vi "Update Online Status List.vi"(8 "error in (no error)":errorcluster, 10 "Online Status List":string[](array[string]), 11 "Chat Window Controller UI in":refnum<class "Chat Window Controller UI.lvclass">) -> (0 "error out":errorcluster, 3 "Chat Window Controller UI out":refnum<class "Chat Window Controller UI.lvclass">)   [LabVIEW 2020, in "Chat Window UI.lvlib" / "Chat Window Controller UI.lvclass"]
uses:
  Chat Window Controller UI.lvclass
  Chat Window Controller UI.lvclass/Chat Window Controller UI.ctl
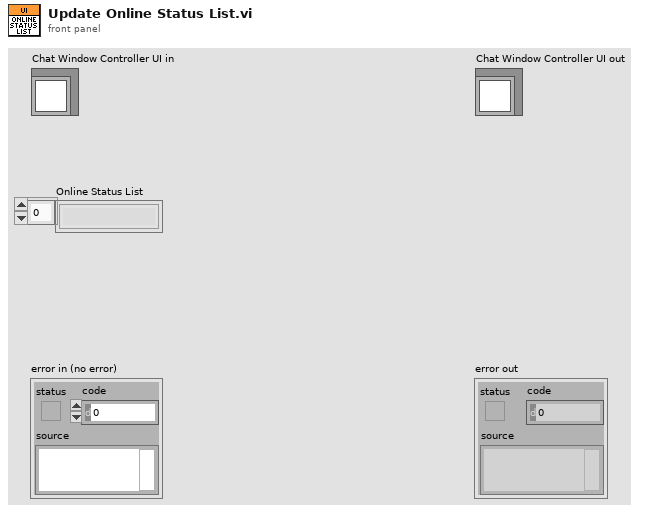
[diagram p1: front panel]
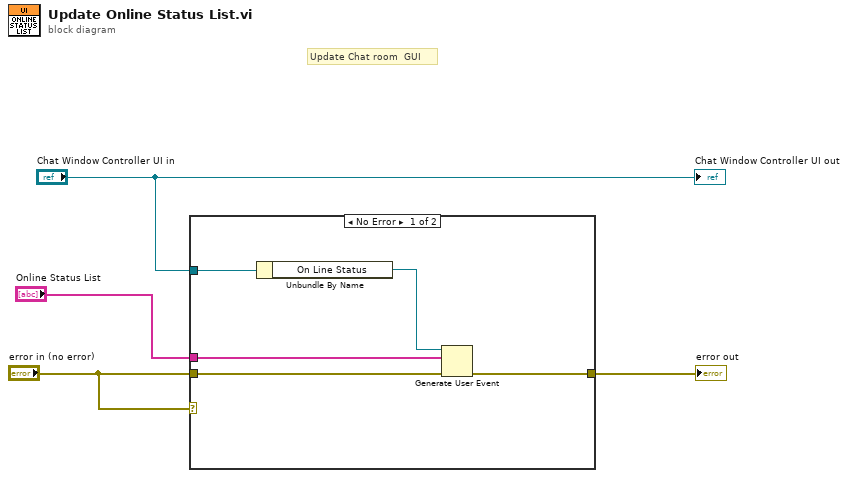
[diagram p0: block diagram]
diagram:
  # "Update Chat room  GUI"
  n1 = case shown="No Error" "error in (no error)" {
    tunnel: "error in (no error)" -> [w8 w10]
    tunnel: [w7 w10] -> w4
    tunnel: "Chat Window Controller UI in" -> [w6 _]
    tunnel: "Online Status List" -> [w5 _]
    frame No Error {
      n2 = Unbundle By Name(w6) -> ("On Line Status"=w9:refnum<user-event>)
      n3 = Generate User Event(user event=w9, event data cluster=w5, error in=w8) -> (error out=w7:errorcluster)  [unwired: 1 in, 1 out]
    }
    frame Error {
    }
  }
  "error out" <- w4
  "Chat Window Controller UI out" <- "Chat Window Controller UI in"
